vi "Get IO Status String.vi"(10 "Loop Index":i32, 11 "Error Status":bool) -> (3 "Output String":string)   [LabVIEW 2018, in "Outputs.lvlib"]
doc: "Converts a boolean error status to a string for logging purpooses. If error, output 0, if not error, outputs 1. Every iteration of 4, inserts a comma before the 0 or 1."
uses:
  Outputs.lvlib
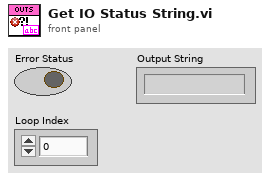
[diagram p1: front panel]
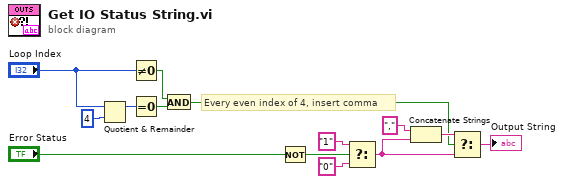
[diagram p0: block diagram]
diagram:
  # "Every even index of 4, insert comma"
  n1 = Quotient & Remainder(x="Loop Index", y=4) -> (x-y*floor(x/y)=w6:i32)  [unwired: 1 out]
  n2 = Not Equal To 0?(x="Loop Index") -> (x != 0?=w2:bool)
  n3 = Equal To 0?(x=w6) -> (x = 0?=w11:bool)
  n4 = And(x=w2, y=w11) -> (x .and. y?=w3:bool)
  n5 = Not(x="Error Status") -> (.not. x?=w7:bool)
  n6 = Select(t="1", s=w7, f="0") -> (s? t:f=w13:string)
  n7 = Concatenate Strings("," ("string"), w13) -> (w12:string)
  n8 = Select(t=w12, s=w3, f=w13) -> (s? t:f=→"Output String":string)
